vi "Cast Sensor Data X5-8.vi"(8 "Map":map{string, dbl}(c390), 9 "Invalid Data":bool[](array[boolean]), 10 "Connected":bool[](array[boolean]), 11 "register values":u16[](array[numeric])) -> (3 "map out":map{string, dbl}(c390))   [LabVIEW 2024, in "IOLink.lvlib"]
uses:
  IOLink.lvlib
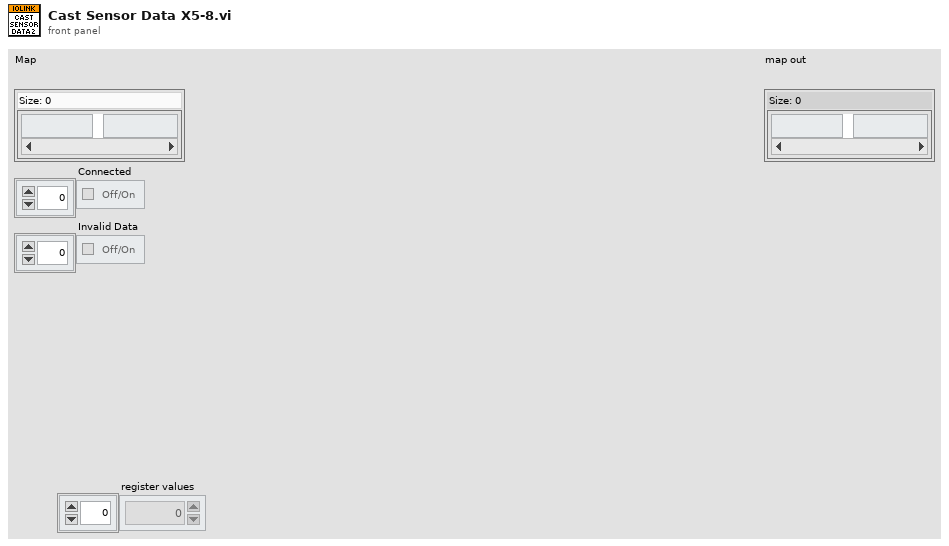
[diagram p1: front panel]
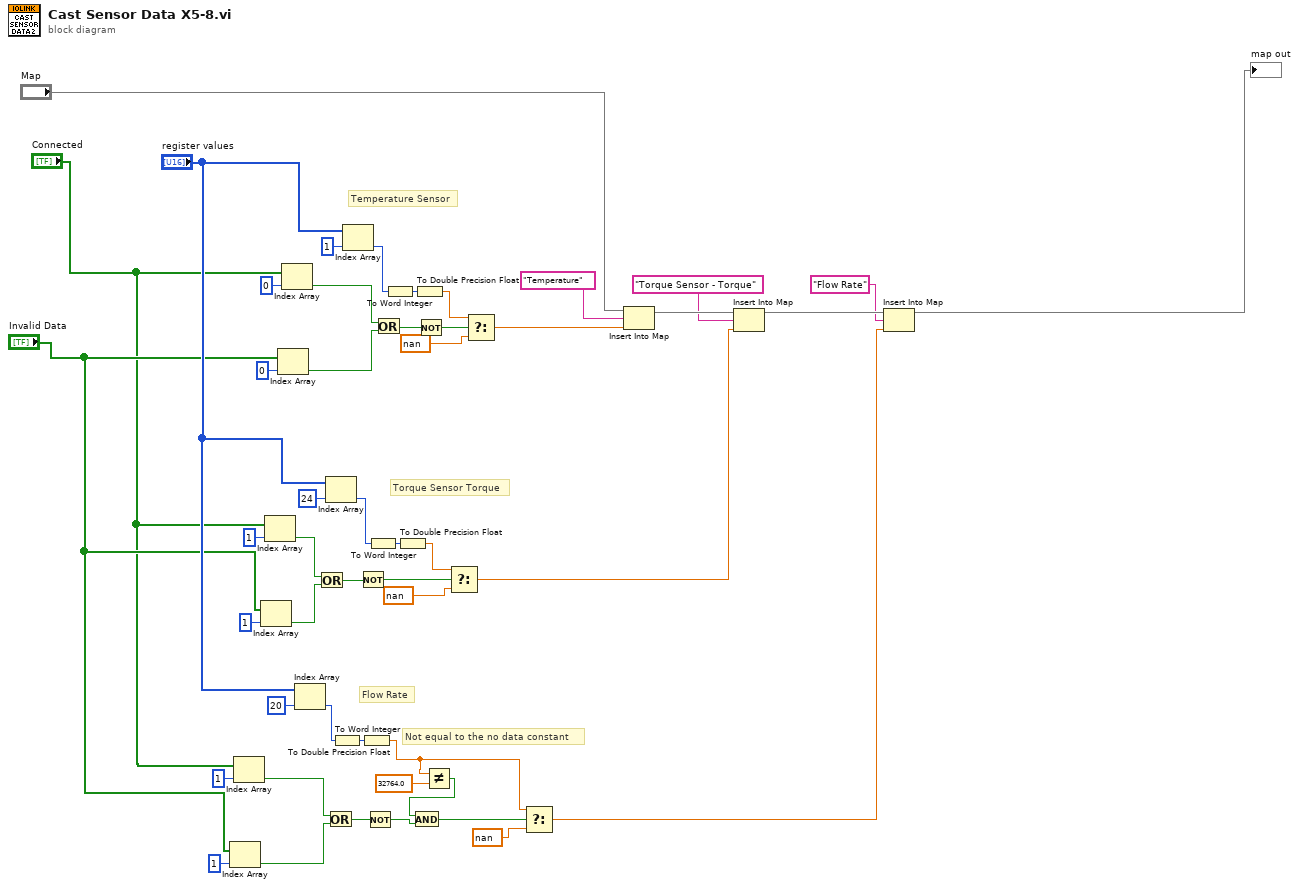
[diagram p0: block diagram]
diagram:
  # "Not equal to the no data constant"
  # "Flow Rate"
  # "Torque Sensor Torque"
  # "Temperature Sensor"
  n1 = Index Array(array="Invalid Data", index=1) -> (element=w30:bool)
  n2 = Index Array(array="Connected", index=1) -> (element=w31:bool)
  n3 = Index Array(array="Invalid Data", index=1) -> (element=w35:bool)
  n4 = Index Array(array="Connected", index=1) -> (element=w34:bool)
  n5 = Index Array(array="Invalid Data", index=0) -> (element=w46:bool)
  n6 = Index Array(array="Connected", index=0) -> (element=w47:bool)
  n7 = Index Array(array="register values", index=20) -> (element=w27:u16)
  n8 = Or(x=w34, y=w35) -> (x .or. y?=w6:bool)
  n9 = Index Array(array="register values", index=24) -> (element=w38:u16)
  n10 = Or(x=w31, y=w30) -> (x .or. y?=w2:bool)
  n11 = To Word Integer(number=w27) -> (16bit integer=w26:i16)
  n12 = Index Array(array="register values", index=1) -> (element=w43:u16)
  n13 = Not(x=w6) -> (.not. x?=w5:bool)
  n14 = To Double Precision Float(number=w26) -> (double precision float=w9:dbl)
  n15 = Not(x=w2) -> (.not. x?=w1:bool)
  n16 = To Word Integer(number=w38) -> (16bit integer=w39:i16)
  n17 = Or(x=w47, y=w46) -> (x .or. y?=w4:bool)
  n18 = To Word Integer(number=w43) -> (16bit integer=w42:i16)
  n19 = To Double Precision Float(number=w39) -> (double precision float=w40:dbl)
  n20 = To Double Precision Float(number=w42) -> (double precision float=w41:dbl)
  n21 = Not(x=w4) -> (.not. x?=w3:bool)
  n22 = Not Equal?(x=w9, y=32764.0) -> (x != y?=w8:bool)
  n23 = And(x=w8, y=w1) -> (x .and. y?=w7:bool)
  n24 = Select(t=w40, s=w5, f=nan) -> (s? t:f=w19:dbl)
  n25 = Select(t=w41, s=w3, f=nan) -> (s? t:f=w22:dbl)
  n26 = Select(t=w9, s=w7, f=nan) -> (s? t:f=w16:dbl)
  n27 = Insert Into Map(map in="Map", key="Temperature", value=w22) -> (map out=w21:map{string, dbl})  [unwired: 2 out]
  n28 = Insert Into Map(map in=w21, key="Torque Sensor - Torque", value=w19) -> (map out=w18:map{string, dbl})  [unwired: 2 out]
  n29 = Insert Into Map(map in=w18, key="Flow Rate", value=w16) -> (map out=→"map out":map{string, dbl})  [unwired: 2 out]
